vi "Configure Output.vi"(7 "Enable Output (T: Enable)":bool=TRUE, 8 "error in (no error)":errorcluster, 9 "Voltage Level (0.0 V)":dbl format="%.3g", 10 "Channel (1: Channel 1)":i32(ring)=1 items=["Channel 1"=1, "Channel 2"=2, "Channel 3"=3], 11 "VISA resource name":refnum<visa-resource-name>) -> (0 "error out":errorcluster, 3 "VISA resource name out":refnum<visa-resource-name>)   [LabVIEW 2020, in "Agilent E363X Series.lvlib"]
doc: "Configures the power supply's output voltage level, channel, voltage range, and enables or disables the output."
uses:
  Agilent E363X Series.lvlib
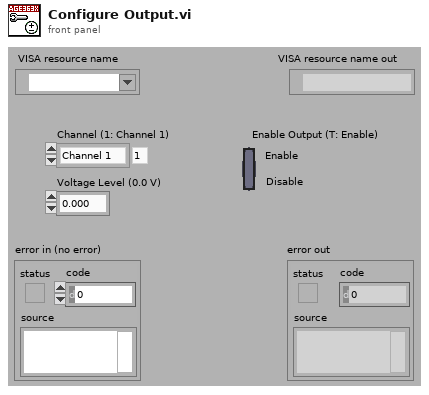
[diagram p1: front panel]
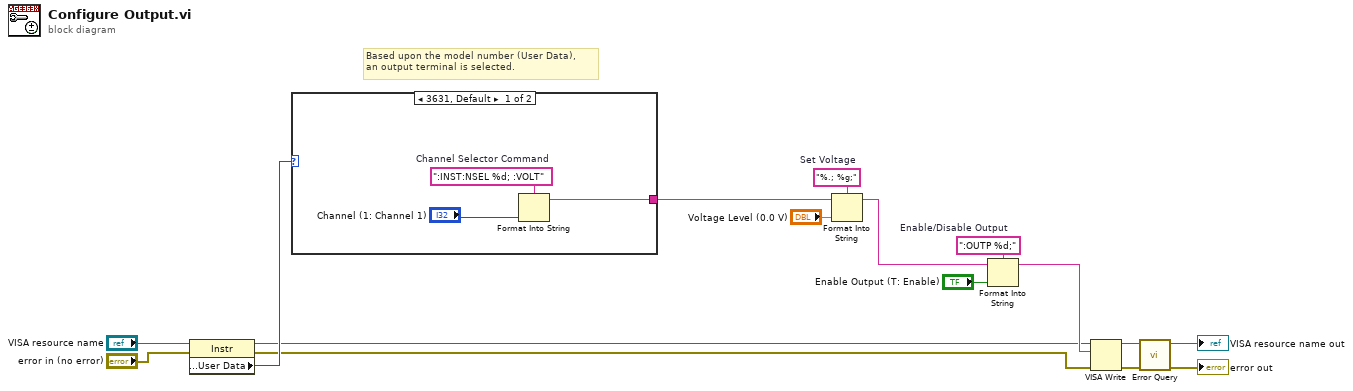
[diagram p0: block diagram]
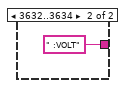
[diagram p2: hidden frame]
diagram:
  w11 = ":OUTP %d;"  # Enable/Disable Output
  w12 = "%.; %g;"  # Set Voltage
  # "Based upon the model number (User Data), \nan output terminal is selected."
  n1 = property on="Property Node" class="Instr"(reference="VISA resource name", error in="error in (no error)") -> (reference out=w4:refnum<visa-resource-name>, error out=w2:errorcluster, "General Settings:User Data"=w6:u32)
  n2 = case shown="3631, Default" w6 {
    tunnel: [w18 " :VOLT" ("Range Selector Command")] -> w1
    frame 3631, Default {
      w19 = ":INST:NSEL %d; :VOLT"  # Channel Selector Command
      n3 = Format Into String(format string=w19, "Channel (1: Channel 1)") -> (resulting string=w18:string)  [unwired: 2 in, 1 out]
    }
    frame 3632..3634 {
    }
  }
  n4 = Format Into String(format string=w12, initial string=w1, "Voltage Level (0.0 V)") -> (resulting string=w7:string)  [unwired: 1 in, 1 out]
  n5 = Format Into String(format string=w11, initial string=w7, "Enable Output (T: Enable)") -> (resulting string=w8:string)  [unwired: 1 in, 1 out]
  n6 = VISA Write(VISA resource name=w4, write buffer=w8, error in (no error)=w2) -> (VISA resource name out=w10:refnum<visa-resource-name>, error out=w9:errorcluster)  [unwired: 1 out]
  n7 = call "Error Query.vi"("error in (no error)"=w9, "VISA resource name"=w10) -> ("error out"=→"error out":errorcluster, "VISA resource name out"=→"VISA resource name out":refnum<visa-resource-name>)  [unwired: 6 in, 2 out]
